vi "Database-ActorMain.vi"(0 "FTW Actor Instance Configuration":T1="{\n  \"Identity\": \"ActorName\",\n  \"InboxAddress\": \"tcp://127.0.0.1:*\",\n  \"PublisherAddress\": \"tcp://127.0.0.1:*\",\n  \"DebugEnableInboxLogging\": false,\n  \"DebugEnableJobLogging\": false,\n  \"DebugShowPanel\": false\n}", 11 "error in":errorcluster) -> (15 "error out":errorcluster)   [LabVIEW 2013, in "Database-Actor.lvclass"]
uses:
  Database-Actor.lvclass
  ftw-dataflow/Actor/src/Utility/FTW-Actor-Configuration.ctl
  Database-Actor.lvclass/Database-Actor.ctl
  ftw-dataflow/Core/src/JSON/FTW-JSON-RegexParse.vi
  ftw-dataflow/Core/src/Error/FTW-ERR-ThrowGenericError.vi
  ftw-dataflow/Core/src/Container/FTW-Container-Construct.vi
  ftw-dataflow/Core/src/Container/FTW-Container-Load-JSON.vi
  ftw-dataflow/Core/src/Container/FTW-Container-Destroy.vi
  ftw-dataflow/Core/utils/CodeGen/JSON Deserialize/FTW-JSON-Deserialize.xnode
  ftw-dataflow/Actor/src/Instance/FTW-ActorInstance.lvclass
  ftw-dataflow/Actor/src/Message/Request/FTW-Message-IncomingRequest.lvclass
  ITS ERP System/ERP-Container/ERP-ConfigPageNewFeather/ERP-ConfigPageNF.lvclass
  ftw-dataflow/Actor/src/FTW-Actor.lvlib
  ftw-dataflow/Core/src/Container/FTW-Container.lvclass
panel:
  out "Timed out?":bool
  # "Inputs"
  # "Outputs"
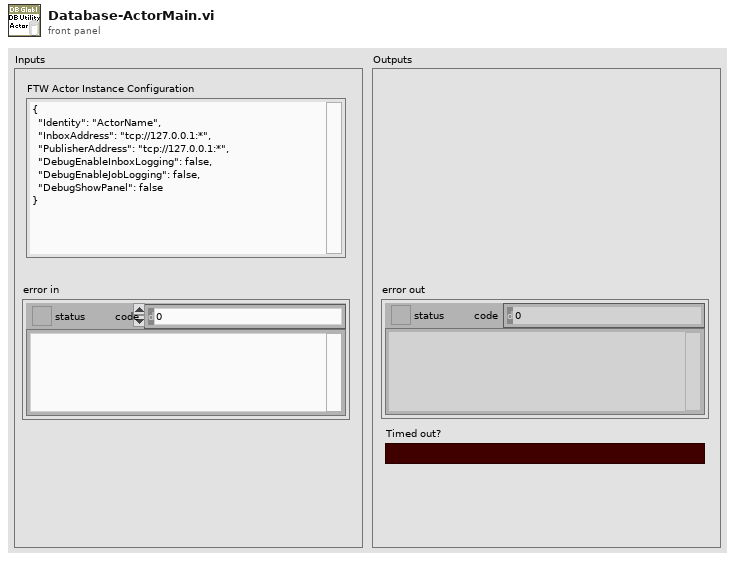
[diagram p1: front panel]
types:
  T1 = typedef "FTW-Actor.lvlib/FTW-Actor-Configuration.ctl" = string
  T2 = cluster{"Incoming Requests":refnum<event-registration>, "Additional Registration Types":refnum<event-registration>}
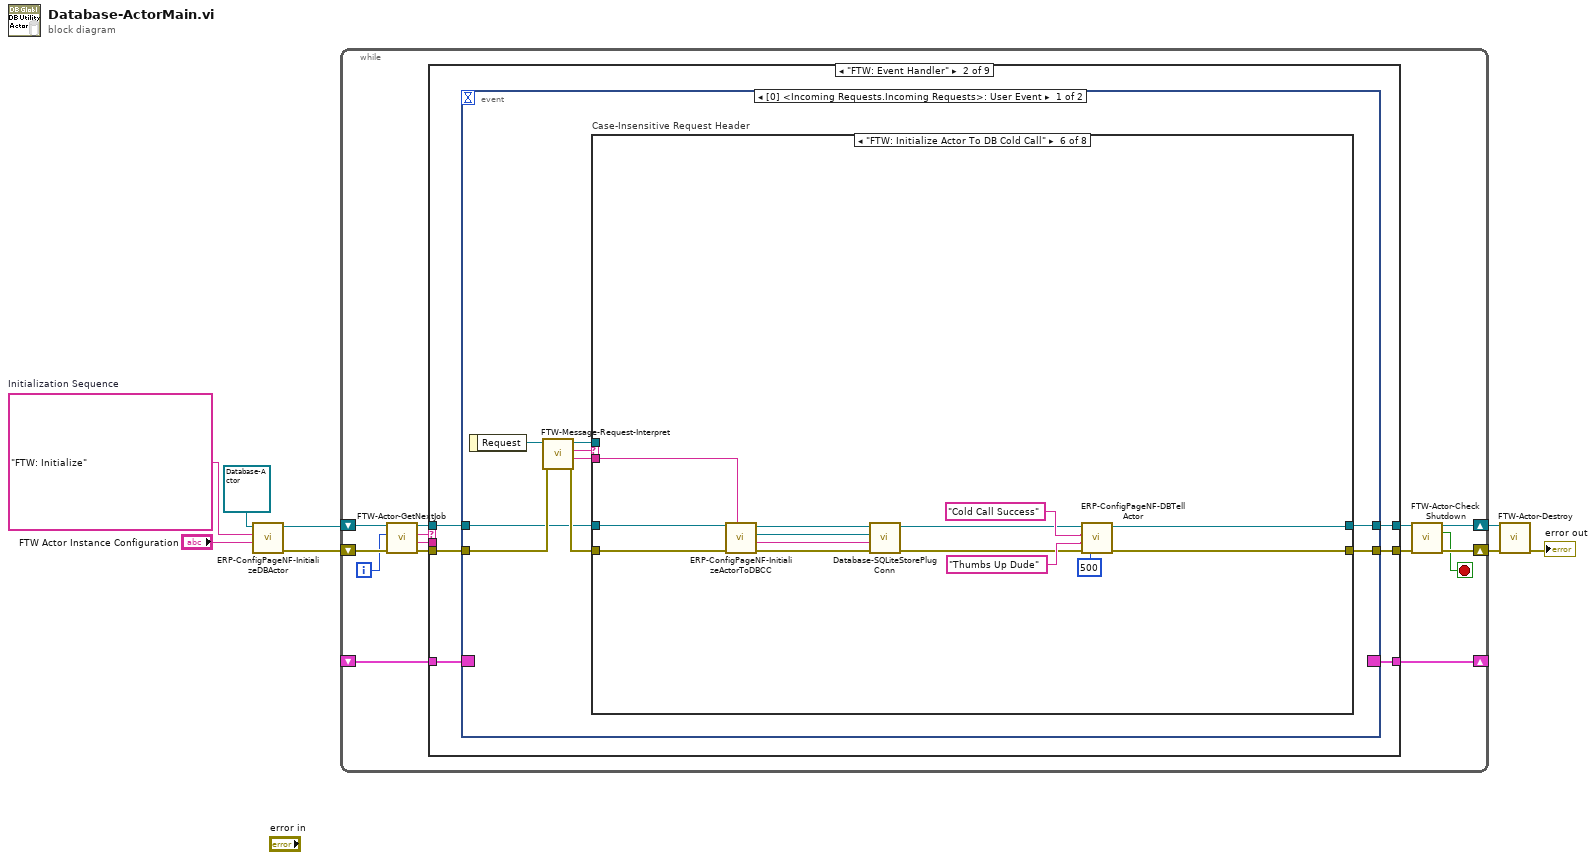
[diagram p0: block diagram]
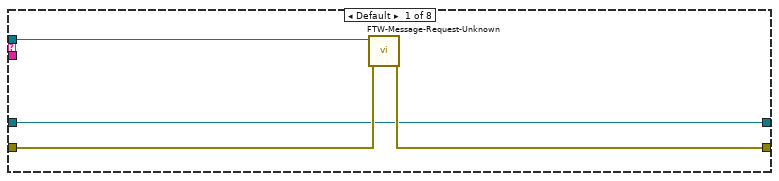
[diagram p3: hidden frame]
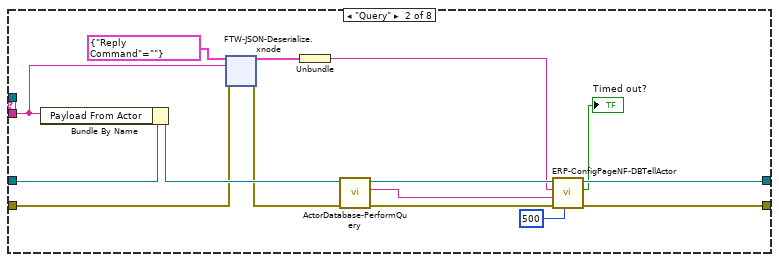
[diagram p4: hidden frame]
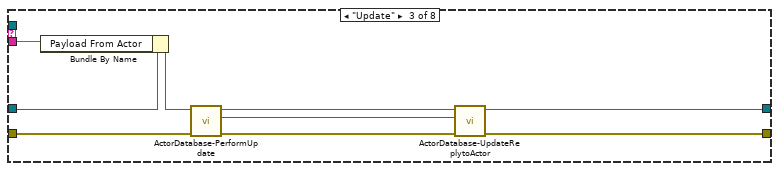
[diagram p5: hidden frame]
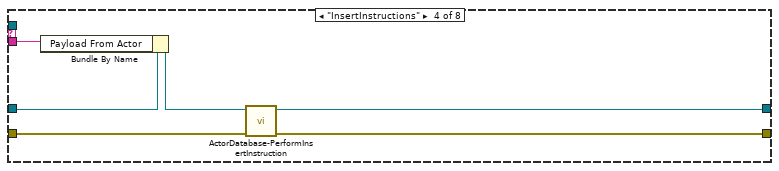
[diagram p6: hidden frame]
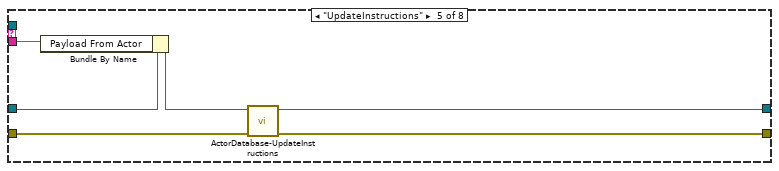
[diagram p7: hidden frame]
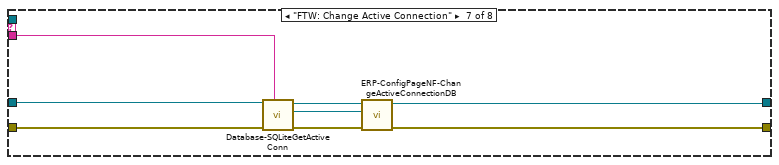
[diagram p8: hidden frame]
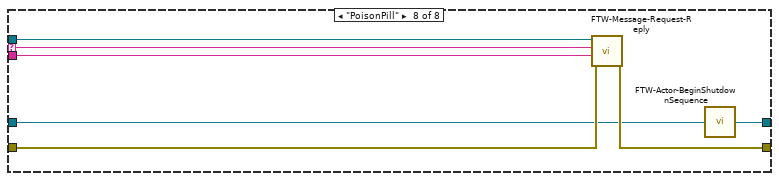
[diagram p9: hidden frame]
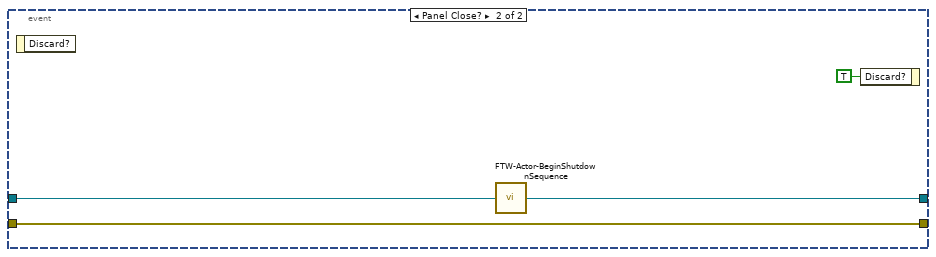
[diagram p10: hidden frame]
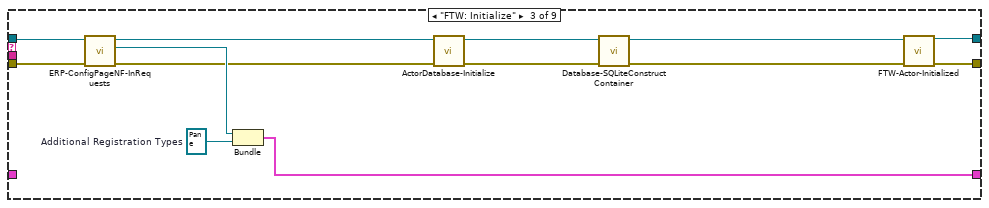
[diagram p11: hidden frame]
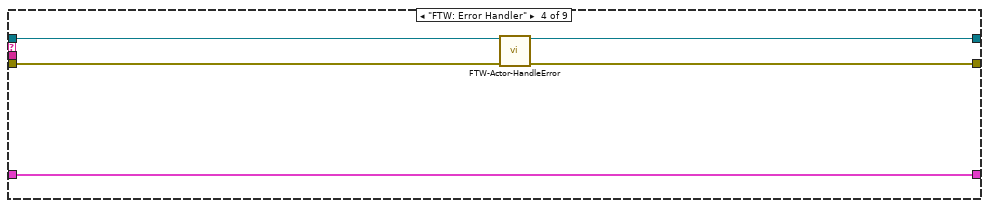
[diagram p12: hidden frame]
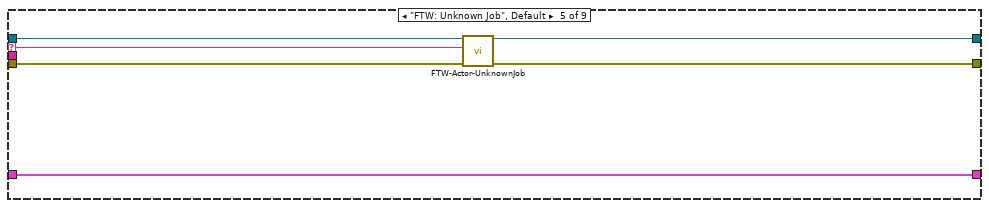
[diagram p13: hidden frame]
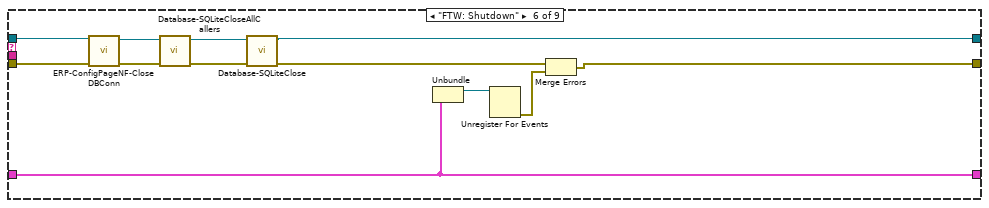
[diagram p14: hidden frame]
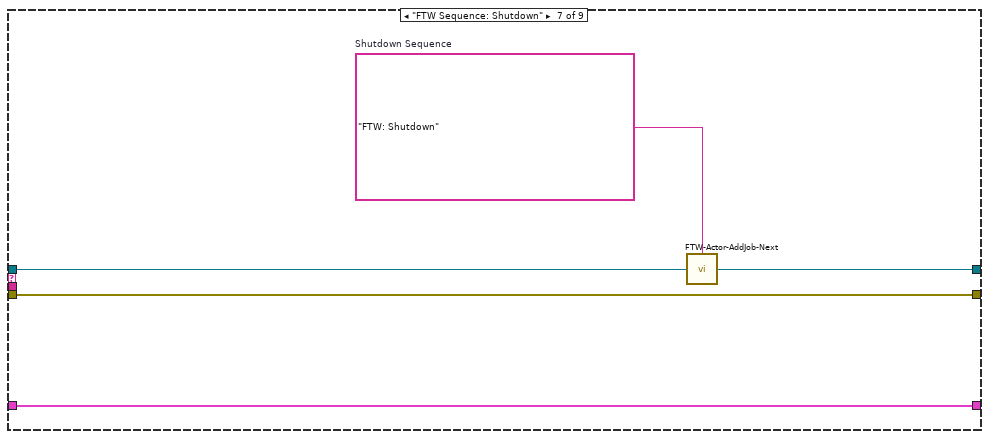
[diagram p15: hidden frame]
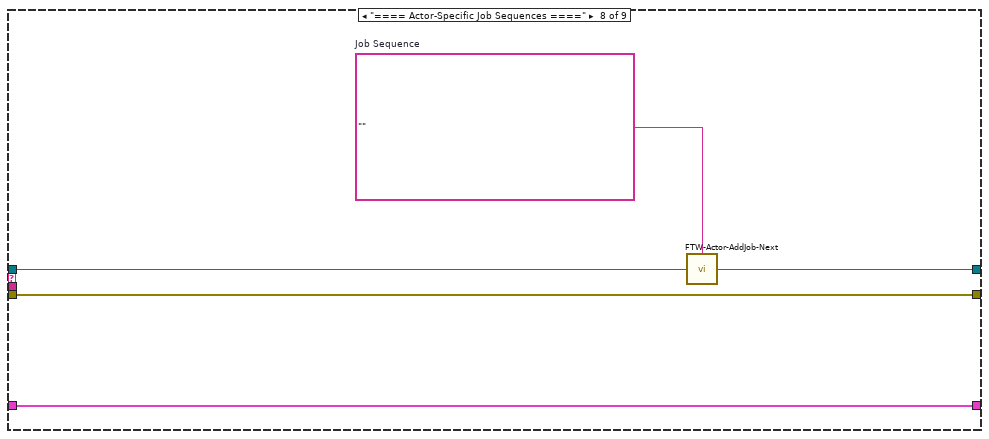
[diagram p16: hidden frame]
diagram:
  w4 = "FTW: Initialize"  # Initialization Sequence
  n1 = call-dynamic "ERP-ConfigPageNF-InitializeDBActor.vi"("FTW Actor Instance Configuration"="FTW Actor Instance Configuration", "Initialization Job Sequence"=w4, "ERP-ConfigPageNF.lvclass"=refnum<class "Database-Actor.lvclass"> refnum ("Database-Actor.lvclass")) -> ("error out"=w6:errorcluster, "ERP-ConfigPageNF out"=w3:refnum<class "Database-Actor.lvclass">)  [unwired: 7 in]
  n2 = while {
    shift-right: [w12] -> w7
    shift-left: w6 -> [w19]
    shift-right: [w9] -> _
    shift-left: _ -> [w22]
    shift-right: [w14] -> w8
    shift-left: w3 -> [w21]
    i -> [w10]
    stop <- w11 stop-if-true
    n3 = call "FTW-Actor-GetNextJob.vi"("error in"=w19, "Jobs Performed"=w10, "FTW Actor Instance"=w21) -> ("error out"=w18:errorcluster, "Job Data"=w16:string, "Job Name"=w17:string, "FTW Actor Instance out"=w20:refnum<class "Database-Actor.lvclass">)  [unwired: 5 in]
    n4 = case shown="\"FTW: Event Handler\"" w17 {
      selector: w17 -> [_ _ _ _ w165 _ _ _ _]
      tunnel: [w24 w31 w154 w160 w168 w180 w186 w191 w195] -> w13
      tunnel: w18 -> [w24 w30 w159 w162 w169 w177 w186 w191 w195]
      tunnel: w22 -> [w25 w26 _ w164 w170 w182 w187 w192 w194]
      tunnel: [w25 w29 w156 w164 w170 w182 w187 w192 w194] -> w9
      tunnel: w16 -> [_ _ _ _ _ _ _ _ _]
      tunnel: [w23 w28 w155 w161 w166 w172 w184 w189 w193] -> w15
      tunnel: w20 -> [w23 w27 w153 w163 w167 w178 w185 w190 w193]
      frame "==== Featherweight Framework Jobs ====" {
      }
      frame "FTW: Event Handler" {
        n5 = event shown="[0] <Incoming Requests.Incoming Requests>: User Event" {
          selector: w26 -> [_ _]
          dyn-events: [_ _] -> w29
          timeout: _ -> [_ _]
          tunnel: [w37 w145] -> w31
          tunnel: w30 -> [w38 w145]
          tunnel: [w36 w143] -> w28
          tunnel: w27 -> [w35 w144]
          event User Event {
            n6 = event-data() -> ("Request"=w39:refnum<class "FTW-Message-IncomingRequest.lvclass">)  [unwired: 1 in]
            n7 = call "FTW-Message-Request-Interpret.vi"("error in"=w38, "FTW Incoming Request"=w39) -> ("error out"=w40:errorcluster, "Request Body"=w33:string, "Request Header"=w34:string, "FTW Incoming Request out"=w32:refnum<class "FTW-Message-IncomingRequest.lvclass">)  [unwired: 6 in]
            n8 = case "Case-Insensitive Request Header" shown="\"FTW: Initialize Actor To DB Cold Call\"" w34 {
              selector: w34 -> [_ _ _ _ _ _ _ w138]
              tunnel: [w43 w55 w93 w102 w108 w123 w129 w139] -> w37
              tunnel: w40 -> [w44 w50 w98 w104 w109 w126 w134 w140]
              tunnel: [w41 w57 w94 w103 w110 w124 w128 w142] -> w36
              tunnel: w35 -> [w41 w58 w100 w106 w112 w127 w135 w136]
              tunnel: w33 -> [_ w48 w101 w107 w113 w125 w133 w137]
              tunnel: w32 -> [w42 _ _ _ _ _ _ w141]
              frame Default {
                n9 = call "FTW-Message-Request-Unknown.vi"("error in"=w44, "FTW Incoming Request"=w42) -> ("error out"=w43:errorcluster)  [unwired: 9 in]
              }
              frame "Query" {
                n10 = Bundle By Name(cluster=w58, "Payload From Actor"=w48) -> (w59:refnum<class "Database-Actor.lvclass">)
                n11 = xnode "FTW-JSON-Deserialize.xnode"("Data Type and Default Values"=cluster{"Reply Command":T1} {"Reply Command"=""}, "JSON String"=w48, "error in"=w50) -> ("Populated Values"=w46:cluster{"Reply Command":T1}, "error out"=w49:errorcluster)
                n12 = Unbundle(w46) -> ("Reply Command"=w45:T1)
                n13 = call "ActorDatabase-PerformQuery.vi"("error in (no error)"=w49, "Database-Actor in"=w59) -> ("error out"=w56:errorcluster, "Payload To Actor"=w54:string, "Database-Actor out"=w51:refnum<class "Database-Actor.lvclass">)  [unwired: 7 in]
                n14 = call "ERP-ConfigPageNF-DBTellActor.vi"("Timeout"=500, "error in (no error)"=w56, "Message Body"=w54, "Message Header"=w45, "ERP-ConfigPageNF in"=w51) -> ("error out"=w55:errorcluster, "Timed out?"=→"Timed out?":bool, "ERP-ConfigPageNF out"=w57:refnum<class "Database-Actor.lvclass">)  [unwired: 4 in]
              }
              frame "Update" {
                n15 = Bundle By Name(cluster=w100, "Payload From Actor"=w101) -> (w99:refnum<class "Database-Actor.lvclass">)
                n16 = call "ActorDatabase-PerformUpdate.vi"("error in (no error)"=w98, "Database-Actor in"=w99) -> ("error out"=w96:errorcluster, "Update Successful"=w95:bool, "Database-Actor out"=w97:refnum<class "Database-Actor.lvclass">)  [unwired: 7 in]
                n17 = call "ActorDatabase-UpdateReplytoActor.vi"("error in (no error)"=w96, "Update Successful"=w95, "Database-Actor in"=w97) -> ("error out"=w93:errorcluster, "Database-Actor out"=w94:refnum<class "Database-Actor.lvclass">)  [unwired: 7 in]
              }
              frame "InsertInstructions" {
                n18 = Bundle By Name(cluster=w106, "Payload From Actor"=w107) -> (w105:refnum<class "Database-Actor.lvclass">)
                n19 = call "ActorDatabase-PerformInsertInstruction.vi"("error in (no error)"=w104, "Database-Actor in"=w105) -> ("error out"=w102:errorcluster, "Database-Actor out"=w103:refnum<class "Database-Actor.lvclass">)  [unwired: 8 in]
              }
              frame "UpdateInstructions" {
                n20 = Bundle By Name(cluster=w112, "Payload From Actor"=w113) -> (w111:refnum<class "Database-Actor.lvclass">)
                n21 = call "ActorDatabase-UpdateInstructions.vi"("error in (no error)"=w109, "Database-Actor in"=w111) -> ("error out"=w108:errorcluster, "Database-Actor out"=w110:refnum<class "Database-Actor.lvclass">)  [unwired: 8 in]
              }
              frame "FTW: Initialize Actor To DB Cold Call" {
                n22 = call "ERP-ConfigPageNF-InitializeActorToDBCC.vi"("JSON String"=w125, "error in (no error)"=w126, "ERP-ConfigPageNF in"=w127) -> ("error out"=w115:errorcluster, "Actor PageID"=w116:T1, "Plugin Caller Ref"=w117:refnum<class "FTW-ActorConnector.lvclass">, "ERP-ConfigPageNF out"=w119:refnum<class "Database-Actor.lvclass">)  [unwired: 5 in]
                n23 = call "Database-SQLiteStorePlugConn.vi"("error in (no error)"=w115, "ActorID"=w116, "FTW Actor Connector"=w117, "Database-Actor in"=w119) -> ("error out"=w114:errorcluster, "Database-Actor out"=w118:refnum<class "Database-Actor.lvclass">)  [unwired: 6 in]
                n24 = call "ERP-ConfigPageNF-DBTellActor.vi"("Timeout"=500, "error in (no error)"=w114, "Message Body"="Thumbs Up Dude", "Message Header"="Cold Call Success", "ERP-ConfigPageNF in"=w118) -> ("error out"=w123:errorcluster, "ERP-ConfigPageNF out"=w124:refnum<class "Database-Actor.lvclass">)  [unwired: 4 in, 1 out]
              }
              frame "FTW: Change Active Connection" {
                n25 = call "Database-SQLiteGetActiveConn.vi"("PageID"=w133, "error in (no error)"=w134, "Database-Actor in"=w135) -> ("error out"=w132:errorcluster, "Active Plugin Caller"=w131:refnum<class "FTW-ActorConnector.lvclass">, "Database-Actor out"=w130:refnum<class "Database-Actor.lvclass">)  [unwired: 6 in]
                n26 = call "ERP-ConfigPageNF-ChangeActiveConnectionDB.vi"("error in (no error)"=w132, "Plugin Caller"=w131, "ERP-ConfigPageNF in"=w130) -> ("error out"=w129:errorcluster, "ERP-ConfigPageNF out"=w128:refnum<class "Database-Actor.lvclass">)  [unwired: 7 in]
              }
              frame "PoisonPill" {
                n27 = call "FTW-Message-Request-Reply.vi"("error in"=w140, "Response Body"=w137, "Response Header"=w138, "FTW Incoming Request"=w141) -> ("error out"=w139:errorcluster)  [unwired: 6 in, 1 out]
                n28 = call "FTW-Actor-BeginShutdownSequence.vi"("FTW Actor Instance"=w136) -> ("FTW Actor Instance out"=w142:refnum<class "Database-Actor.lvclass">)  [unwired: 3 in]
              }
            }
          }
          event Panel Close? {
            n29 = event-data() -> ()  [unwired: 1 in, 1 out]
            n30 = call "FTW-Actor-BeginShutdownSequence.vi"("FTW Actor Instance"=w144) -> ("FTW Actor Instance out"=w143:refnum<class "Database-Actor.lvclass">)  [unwired: 3 in]
            n31 = event-data("Discard?"=TRUE) -> ()  [unwired: 1 in, 1 out]
          }
        }
      }
      frame "FTW: Initialize" {
        w158 = refnum<event-registration> refnum  # Additional Registration Types
        n32 = call "ERP-ConfigPageNF-InRequests.vi"("error in (no error)"=w159, "ERP-ConfigPageNF in"=w153) -> ("error out"=w152:errorcluster, "Incoming Requests"=w157:refnum<event-registration>, "ERP-ConfigPageNF out"=w151:refnum<class "Database-Actor.lvclass">)  [unwired: 7 in]
        n33 = Bundle("Incoming Requests"=w157, "Additional Registration Types"=w158) -> (w156:T2)  [unwired: 1 in]
        n34 = call "ActorDatabase-Initialize.vi"("error in (no error)"=w152, "Database-Actor In"=w151) -> ("error out"=w149:errorcluster, "Database-Actor out"=w150:refnum<class "Database-Actor.lvclass">)  [unwired: 8 in]
        n35 = call "Database-SQLiteConstructContainer.vi"("error in (no error)"=w149, "Database-Actor in"=w150) -> ("error out"=w147:errorcluster, "Database-Actor out"=w148:refnum<class "Database-Actor.lvclass">)  [unwired: 8 in]
        n36 = call-dynamic "FTW-Actor-Initialized.vi"("FTW Actor Instance"=w148, "error in"=w147) -> ("FTW Actor Instance out"=w155:refnum<class "Database-Actor.lvclass">, "error out"=w154:errorcluster)  [unwired: 12 in]
      }
      frame "FTW: Error Handler" {
        n37 = call-dynamic "FTW-Actor-HandleError.vi"("FTW Actor Instance"=w163, "error in"=w162) -> ("FTW Actor Instance out"=w161:refnum<class "Database-Actor.lvclass">, "error out"=w160:errorcluster)  [unwired: 11 in, 1 out]
      }
      frame "FTW: Unknown Job", Default {
        n38 = call-dynamic "FTW-Actor-UnknownJob.vi"("FTW Actor Instance"=w167, "Unknown Job"=w165, "error in"=w169) -> ("FTW Actor Instance out"=w166:refnum<class "Database-Actor.lvclass">, "error out"=w168:errorcluster)  [unwired: 11 in]
      }
      frame "FTW: Shutdown" {
        n39 = call "ERP-ConfigPageNF-CloseDBConn.vi"("error in (no error)"=w177, "ERP-ConfigPageNF in"=w178) -> ("error out"=w176:errorcluster, "ERP-ConfigPageNF out"=w175:refnum<class "Database-Actor.lvclass">)  [unwired: 8 in]
        n40 = call "Database-SQLiteCloseAllCallers.vi"("error in (no error)"=w176, "Database-Actor in"=w175) -> ("error out"=w174:errorcluster, "Database-Actor out"=w173:refnum<class "Database-Actor.lvclass">)  [unwired: 8 in]
        n41 = call "Database-SQLiteClose.vi"("error in (no error)"=w174, "Database-Actor in"=w173) -> ("error out"=w171:errorcluster, "Database-Actor out"=w172:refnum<class "Database-Actor.lvclass">)  [unwired: 8 in]
        n42 = Unbundle(w182) -> ("Incoming Requests"=w181:refnum<event-registration>)  [unwired: 1 out]
        n43 = Unregister For Events(event registration refnum=w181) -> (error out=w179:errorcluster)  [unwired: 1 in]
        n44 = Merge Errors(w171, w179) -> (w180:errorcluster)
      }
      frame "FTW Sequence: Shutdown" {
        w183 = "FTW: Shutdown"  # Shutdown Sequence
        n45 = call "FTW-Actor-AddJob-Next.vi"("Add Next in Job Queue"=w183, "FTW Actor Instance"=w185) -> ("FTW Actor Instance out"=w184:refnum<class "Database-Actor.lvclass">)  [unwired: 2 in]
      }
      frame "==== Actor-Specific Job Sequences ====" {
        w188 = ""  # Job Sequence
        n46 = call "FTW-Actor-AddJob-Next.vi"("Add Next in Job Queue"=w188, "FTW Actor Instance"=w190) -> ("FTW Actor Instance out"=w189:refnum<class "Database-Actor.lvclass">)  [unwired: 2 in]
      }
      frame "==== Actor-Specific Jobs ====" {
      }
    }
    n47 = call "FTW-Actor-CheckShutdown.vi"("FTW Actor Instance"=w15, "error in"=w13) -> ("FTW Actor Instance out"=w14:refnum<class "Database-Actor.lvclass">, "Shutdown?"=w11:bool, "error out"=w12:errorcluster)  [unwired: 11 in]
  }
  n48 = call-dynamic "FTW-Actor-Destroy.vi"("FTW Actor Instance"=w8, "error in"=w7) -> ("error out"=→"error out":errorcluster)  [unwired: 13 in]
